vi "dome_logEvent_AppliedSettingsMatchStart.vi"(8 "error in (no error)":errorcluster, 11 "logevent_AppliedSettingsMatchStart_Ctl":T1) -> (0 "error out":errorcluster, 2 "function return":i32, 3 "logevent_AppliedSettingsMatchStart_Ctl out":T1)   [LabVIEW 2016, in "SALLV_dome.lvlib"]
doc: "int dome_shm_logEvent_AppliedSettingsMatchStartLV(dome_logevent_AppliedSettingsMatchStartLV *logevent_AppliedSettingsMatchStart_Ctl );"
uses:
  SALLV_dome.lvlib
  DataTypes/logevent_AppliedSettingsMatchStart.ctl
  SALLV_dome.so
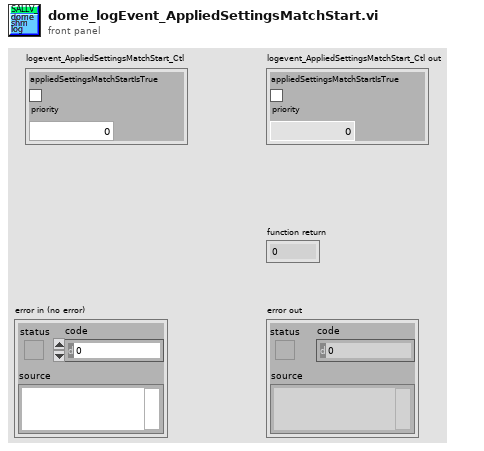
[diagram p1: front panel]
types:
  T1 = typedef "SALLV_dome.lvlib/logevent_AppliedSettingsMatchStart.ctl" = cluster{"appliedSettingsMatchStartIsTrue":bool, "priority":i32}
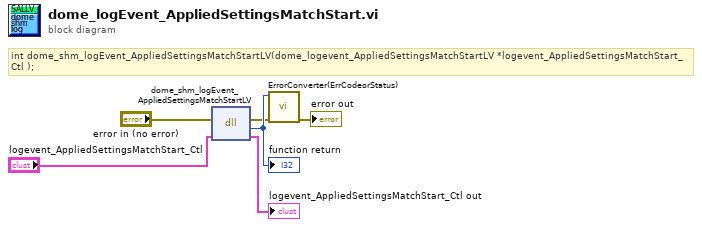
[diagram p0: block diagram]
diagram:
  # "int dome_shm_logEvent_AppliedSettingsMatchStartLV(dome_logevent_AppliedSettingsMatchStartLV *logevent_AppliedSettingsMatchStart_Ctl );"
  n1 = dll-call lib="home/andres/Desktop/SALLV_dome/SALLV_dome.*" fn="dome_shm_logEvent_AppliedSettingsMatchStartLV"(error in="error in (no error)", "logevent_AppliedSettingsMatchStart_Ctl"="logevent_AppliedSettingsMatchStart_Ctl") -> (error out=w2:errorcluster, w6:i32, "logevent_AppliedSettingsMatchStart_Ctl"=→"logevent_AppliedSettingsMatchStart_Ctl out":T1)  [unwired: 2 in, 1 out]
  "function return" <- w6
  n2 = call "ErrorConverter(ErrCodeorStatus).vi"("error in (no error)"=w2, "error code"=w6) -> ("error out"=→"error out":errorcluster)  [unwired: 9 in]
